vi "Set Edge Trigger.vi"(6 "Trigger Slope (0: Rising)":u16(ring) items=["Rising", "Falling", "Either"], 7 "Trigger Coupling (0 : DC)":u16(ring) items=["DC", "HF Reject", "LF Reject", "Noise Reject", "AC"], 8 "error in (no error)":errorcluster, 9 "Trigger Level (0.0 V)":dbl, 10 "Analog Channel":T1, 11 "PicoScope 3000a in":refnum<class "PicoScope 3000a.lvclass">) -> (0 "error out":errorcluster, 3 "PicoScope 3000a out":refnum<class "PicoScope 3000a.lvclass">)   [LabVIEW 2018, in "PicoScope 3000a.lvlib" / "PicoScope 3000a.lvclass"]
uses:
  PicoScope 3000a.lvclass
  PPLs/Oscilloscope/Parent/Oscilloscope.lvlibp/Custom Controls/Analog Channels.ctl
  PicoScope 3000a.lvclass/PicoScope 3000a.ctl
  ps3000a.dll
  <instrlib>/PicoScope/PicoScope.lvlib
  PPLs/Oscilloscope/Parent/Oscilloscope.lvlibp
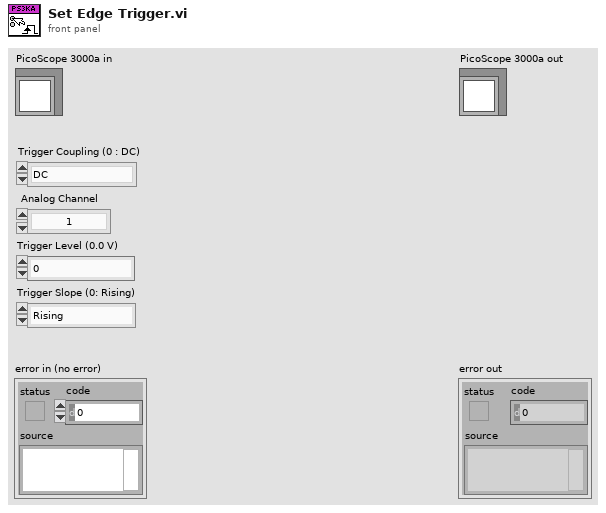
[diagram p1: front panel]
types:
  T1 = typedef "Oscilloscope.lvlibp/Analog Channels.ctl" = enum16{"1", "2", "3", "4", "5", "6", "7", "8", "9", "10", "11", "12", "13", "14", "15", "16"}
  T2 = cluster{"Trigger Slope (0: Rising)":u16, "Analog Channel":T1, "Trigger Level (0.0 V)":dbl, "Trigger Coupling (0 : DC)":u16}
  T3 = cluster{"Trigger Enabled":bool, "Trigger Source":enum32{"Channel A", "Channel B", "Channel C", "Channel D", "Ext."}, "Trigger Threshold (volts)":dbl, "Trigger Direction":u32, "Trigger Delay (samples)":u32, "Auto Trigger Time (ms)":i16}
  T4 = enum32{"Channel A", "Channel B", "Channel C", "Channel D", "Ext."}
  T5 = cluster{"Enabled":bool, "Coupling":u32, "Range":u32, "Analogue Offset":sgl}[]
  T6 = cluster{"Enabled":bool, "Coupling":u32, "Range":u32, "Analogue Offset":sgl}
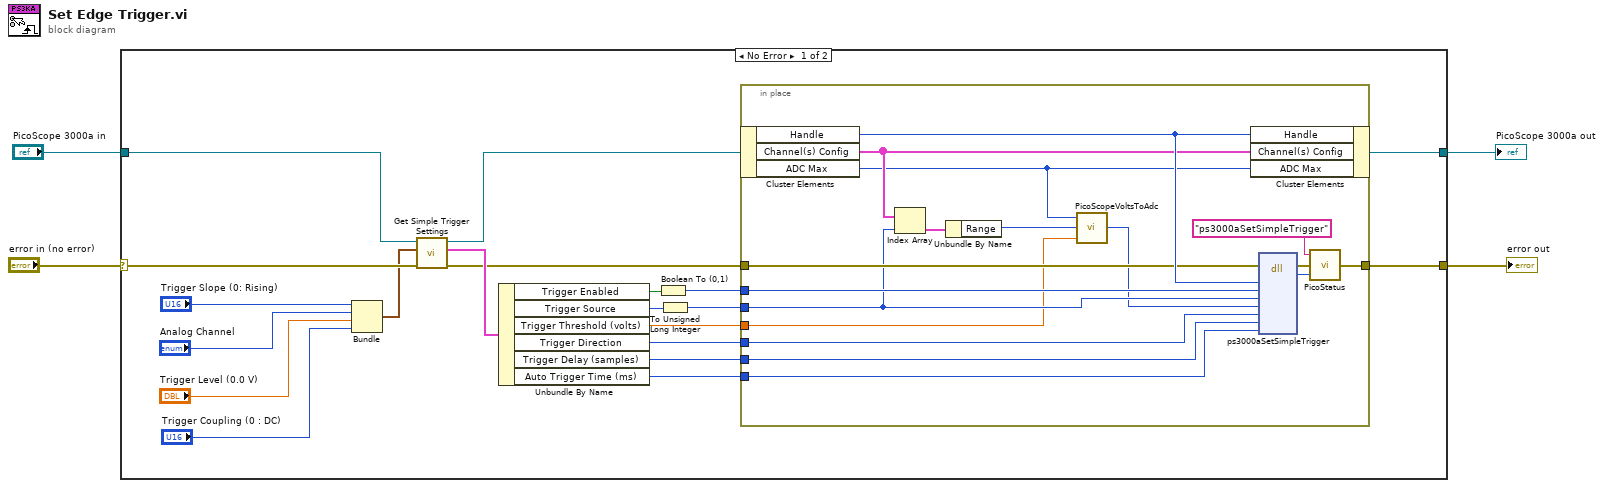
[diagram p0: block diagram]
diagram:
  n1 = case shown="No Error" "error in (no error)" {
    selector: "error in (no error)" -> [w17 w42]
    tunnel: "PicoScope 3000a in" -> [w18 w43]
    tunnel: [w24 w43] -> w2
    tunnel: [w23 w42] -> w1
    frame No Error {
      n2 = Bundle("Trigger Slope (0: Rising)"="Trigger Slope (0: Rising)", "Analog Channel"="Analog Channel", "Trigger Level (0.0 V)"="Trigger Level (0.0 V)", "Trigger Coupling (0 : DC)"="Trigger Coupling (0 : DC)") -> (w15:T2)  [unwired: 1 in]
      n3 = call "Get Simple Trigger Settings.vi"("error in (no error)"=w17, "Edge Trigger Settings"=w15, "PicoScope 3000a in"=w18) -> ("error out"=w7:errorcluster, "Simple Trigger Settings"=w16:T3, "PicoScope 3000a out"=w6:refnum<class "PicoScope 3000a.lvclass">)  [unwired: 6 in]
      n4 = Unbundle By Name(w16) -> ("Trigger Enabled"=w14:bool, "Trigger Source"=w12:T4, "Trigger Threshold (volts)"=w5:dbl, "Trigger Direction"=w10:u32, "Trigger Delay (samples)"=w9:u32, "Auto Trigger Time (ms)"=w8:i16)
      n5 = Boolean To (0,1)(Boolean=w14) -> (0, 1=w13:i16)
      n6 = To Unsigned Long Integer(number=w12) -> (unsigned 32bit integer=w11:u32)
      n7 = in-place {
        in-place-border: w7 -> [w37]
        in-place-border: [w36] -> w23
        in-place-border: w13 -> [w35]
        in-place-border: w11 -> [w31]
        in-place-border: w10 -> [w34]
        in-place-border: w9 -> [w33]
        in-place-border: w8 -> [w32]
        in-place-border: w5 -> [w26]
        n8 = in-place-cluster #1(w6) -> ("Handle"=w38:i16, "Channel(s) Config"=w28:T5, "ADC Max"=w27:i16)
        n9 = Index Array(array=w28, index=w31) -> (element=w30:T6)
        n10 = Unbundle By Name(w30) -> ("Range"=w29:u32)
        n11 = call <instrlib>:"PicoScopeVoltsToAdc.vi"("Max_adc"=w27, "Volts"=w26, "Range Index"=w29) -> ("ADC count"=w25:i16)
        n12 = in-place-cluster #1("Handle"=w38, "Channel(s) Config"=w28, "ADC Max"=w27) -> (w24:refnum<class "PicoScope 3000a.lvclass">)
        n13 = dll-call lib="ps3000a.dll" fn="ps3000aSetSimpleTrigger" ("ps3000.dll:_ps3000_open_unit@0")(error in=w37, "handle"=w38, "enabled"=w35, "source"=w31, "threshold"=w25, "direction"=w34, "delay"=w33, "autoTrigger_ms"=w32) -> (error out=w40:errorcluster, "PICO_STATUS"=w41:u32)  [unwired: 9 in, 1 out]
        n14 = call <instrlib>:"PicoStatus.vi"("PICO STATUS"=w41, "error in"=w40, "source"="ps3000aSetSimpleTrigger") -> ("error out"=w36:errorcluster)
      }
    }
    frame Error {
    }
  }
  "error out" <- w1
  "PicoScope 3000a out" <- w2
